vi "Task2.vi"() -> ()   [LabVIEW 2014, in "Diaz_Excercise_3.lvrbt"]
uses:
  Diaz_Excercise_3.lvrbt
  <vilib>/NXT/Block Support/NXT_InputPort.ctl
  <vilib>/NXT/Block Support/NXT_OutputPort.ctl
  <vilib>/NXT/NXTIO Xnodes/NXTIONodeSubVIs/NXTMoveMotors.vi
  <vilib>/NXT/Subs/LVHSConnector.ctl
  <vilib>/NXT/NXTIO Xnodes/AddressXNode/NXTIOAddress.xnode
  <vilib>/NXT/NXTIO Xnodes/NXTIOXNode/NXTIO.xnode
  <vilib>/NXT/LegoClasses/BrickReference/BrickReference.lvclass
panel:
  in  "stop":bool
  out "distance from wall":dbl
  out "number of loop iterations":i32
  out "final iteration value":i32
  out "current iteration":i32
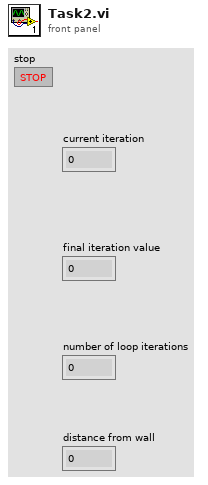
[diagram p1: front panel]
types:
  T1 = typedef "NXT_OutputPort.ctl" = u8
  T2 = typedef "NXT_InputPort.ctl" = u32
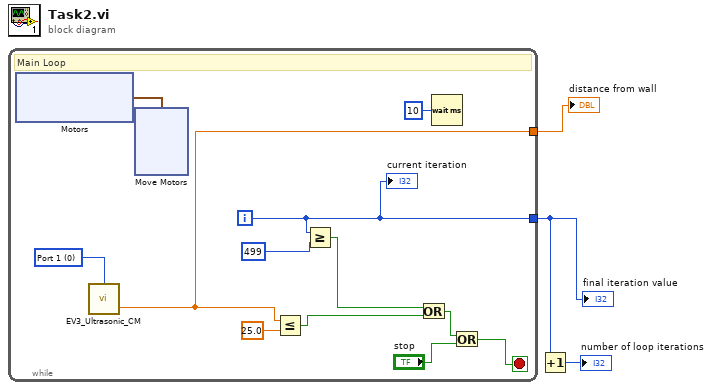
[diagram p0: block diagram]
diagram:
  n1 = while {
    tunnel: [w5] -> w1
    tunnel: [w4] -> w3
    i -> [w5]
    stop <- w11 stop-if-true
    w14 = T2 0 items=["Port 1", "Port 2", "Port 3", "Port 4"] ("Port (Port 1)")
    # "Main Loop"
    n2 = xnode "Motors"() -> ("Motor"=w15:cluster{"Port":T1, "Port":T1})
    n3 = call <vilib>:"EV3_Ultrasonic_CM.vi"("Port (Port 1)"=w14) -> ("Centimeters"=w4:sgl)  [unwired: 2 in, 1 out]
    n4 = xnode "Move Motors"("Motors"=w15) -> ()  [unwired: 3 in, 1 out]
    n5 = Less Or Equal?(x=w4, y=sgl 25.0) -> (x <= y?=w9:bool)
    n6 = Greater Or Equal?(x=w5, y=499) -> (x >= y?=w7:bool)
    n7 = Or(x=w7, y=w9) -> (x .or. y?=w10:bool)
    n8 = Wait (ms)(milliseconds to wait=u32 10) -> ()  [unwired: 1 out]
    n9 = Or(x=w10, y="stop") -> (x .or. y?=w11:bool)
    "current iteration" <- w5
  }
  "distance from wall" <- w3
  "final iteration value" <- w1
  n10 = Increment(x=w1) -> (x+1=→"number of loop iterations":i32)
